vi "Wrap iPerf Test.vi"(7 "DUT Settings Ref":refnum<vi>, 8 "error in":errorcluster, 10 "iPerf Test Parameters":T2={"CLIENT iPERF PORT"=61000, "Protocol"=enum."TCP", "Force traffic (UDP only)"=enum."1M", "DURATION iPERF TEST (s)"=10, "Stack mode"=enum."IP stack"}, 11 "Client_adapter_IP_remote":string) -> (0 "error out":errorcluster, 2 "Server results":T1, 3 "Client results":T1)   [LabVIEW 2026]
uses:
  emea-tra-iPerf_bus_load_test/support/iperf3.Results.ctl
  emea-tra-iPerf_bus_load_test/support/iPerf_parameter.ctl
  emea-tra-iPerf_bus_load_test/support/iPerf_protocol.ctl
  emea-tra-iPerf_bus_load_test/support/bandwidth_selector.ctl
  emea-tra-iPerf_bus_load_test/support/Remote_test_info.ctl
  emea-tra-iPerf_bus_load_test/iPerfTest.lvlib
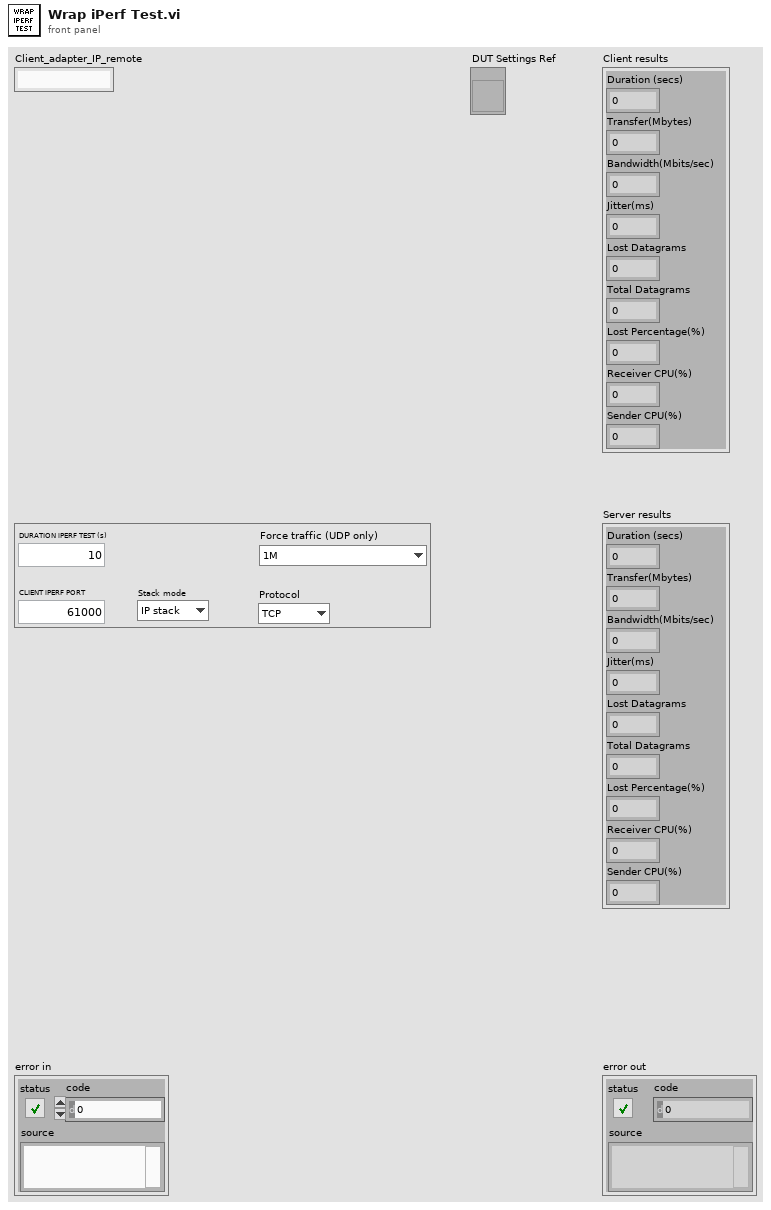
[diagram p1: front panel]
types:
  T1 = typedef "iPerfTest.lvlib/iperf3.Results.ctl" = cluster{"Duration (secs)":dbl, "Transfer(Mbytes)":dbl, "Bandwidth(Mbits/sec)":dbl, "Jitter(ms)":dbl, "Lost Datagrams":i32, "Total Datagrams":i32, "Lost Percentage(%)":dbl, "Receiver CPU(%)":dbl, "Sender CPU(%)":dbl}
  T2 = cluster{"CLIENT iPERF PORT":u16, "Protocol":enum16{"UDP", "TCP"}, "Force traffic (UDP only)":enum16{"1M", "10M", "20M", "30M", "40M", "50M", "100M", "500M", "1000M"}, "DURATION iPERF TEST (s)":u16, "Stack mode":enum16{"OS stack", "IP stack"}}
  T3 = typedef "iPerfTest.lvlib/Remote_test_info.ctl" = cluster{"PuTTY root folder ":path, "Remote Account Username":string, "Remote Account Password":string, "Server_adapter_IP_remote":string, "Client_adapter_IP_remote":string, "iPerf_path_remote_server":path, "iPerf_path_remote_client":path}
  T4 = typedef "iPerf_parameter.ctl" = cluster{"iPerf sending duration":i32, "Protocol":T5, "Force traffic (UDP only)":T6, "Port server":i32, "Port client":i32, "Stack mode":enum16{"OS stack", "IP stack"}}
  T5 = typedef "iPerf_protocol.ctl" = enum16{"UDP", "TCP"}
  T6 = typedef "bandwidth_selector.ctl" = enum16{"1M", "10M", "20M", "30M", "40M", "50M", "100M", "500M", "1000M"}
  T7 = enum16{"1M", "10M", "20M", "30M", "40M", "50M", "100M", "500M", "1000M"}
  T8 = typedef "DUT Info.ctl" = cluster{"DUT IP":string, "DUT Username":string, "DUT Password":string, "DUT SSH PORT":u16, "DUT FWD TEST PORT":u16, "DUT MAC ADDRESS":string}
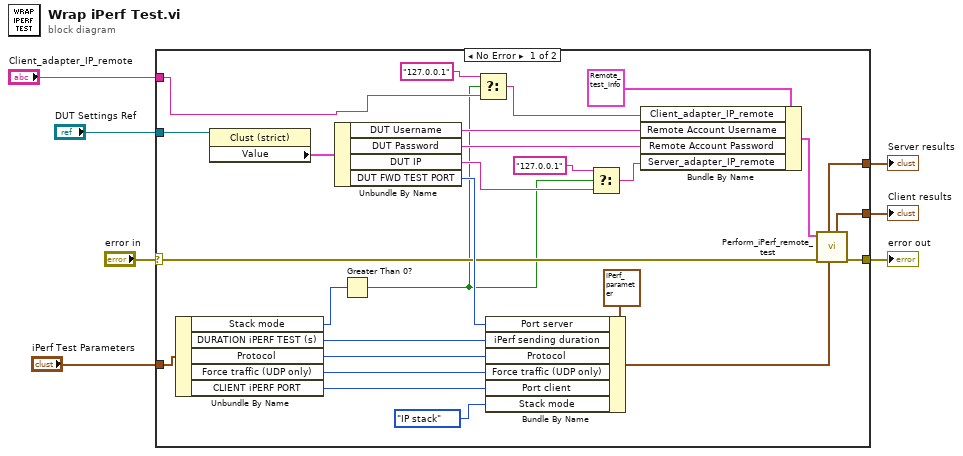
[diagram p0: block diagram]
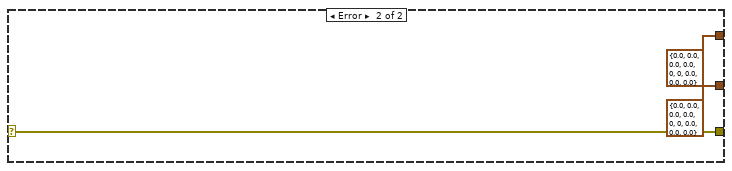
[diagram p2: hidden frame]
diagram:
  n1 = case shown="No Error" "error in" {
    selector: "error in" -> [w16 w35]
    tunnel: [w32 w35] -> w7
    tunnel: "DUT Settings Ref" -> [w30 _]
    tunnel: "iPerf Test Parameters" -> [w26 _]
    tunnel: [w18 T1 {"Duration (secs)"=0.0, "Transfer(Mbytes)"=0.0, "Bandwidth(Mbits/sec)"=0.0, "Jitter(ms)"=0.0, "Lost Datagrams"=0, "Total Datagrams"=0, "Lost Percentage(%)"=0.0, "Receiver CPU(%)"=0.0, "Sender CPU(%)"=0.0} ("Client results")] -> w4
    tunnel: [w17 T1 {"Duration (secs)"=0.0, "Transfer(Mbytes)"=0.0, "Bandwidth(Mbits/sec)"=0.0, "Jitter(ms)"=0.0, "Lost Datagrams"=0, "Total Datagrams"=0, "Lost Percentage(%)"=0.0, "Receiver CPU(%)"=0.0, "Sender CPU(%)"=0.0} ("Server results")] -> w3
    tunnel: "Client_adapter_IP_remote" -> [w10 _]
    frame No Error {
      n2 = Unbundle By Name(w26) -> ("Stack mode"=w12:enum16{"OS stack", "IP stack"}, "DURATION iPERF TEST (s)"=w25:u16, "Protocol"=w24:enum16{"UDP", "TCP"}, "Force traffic (UDP only)"=w23:T7, "CLIENT iPERF PORT"=w20:u16)
      n3 = property class="Clust (strict)"(reference=w30) -> ("Value"=w29:T8)  [unwired: 1 in, 2 out]
      n4 = Unbundle By Name(w29) -> ("DUT Username"=w28:string, "DUT Password"=w27:string, "DUT IP"=w13:string, "DUT FWD TEST PORT"=w22:u16)
      n5 = Greater Than 0?(x=w12) -> (x > 0?=w8:bool)
      n6 = Select(t="127.0.0.1" ("f"), s=w8, f=w10) -> (s? t:f=w9:string)
      n7 = Bundle By Name(cluster=T4 {"iPerf sending duration"=10, "Protocol"=enum."UDP", "Force traffic (UDP only)"=enum."1000M", "Port server"=0, "Port client"=0, "Stack mode"=enum."OS stack"} ("iPerf parameter"), "Port server"=w22, "iPerf sending duration"=w25, "Protocol"=w24, "Force traffic (UDP only)"=w23, "Port client"=w20, "Stack mode"=enum16{"OS stack", "IP stack"}."IP stack") -> (w19:T4)
      n8 = Select(t="127.0.0.1" ("f"), s=w8, f=w13) -> (s? t:f=w15:string)
      n9 = Bundle By Name(cluster=T3 {"PuTTY root folder "=path "C:/dev/emea-tra-iPerf_bus_load_test/utility/Putty_ssh_client", "Remote Account Username"="NI", "Remote Account Password"="123", "Server_adapter_IP_remote"="192.168.178.55", "Client_adapter_IP_remote"="192.168.178.51", "iPerf_path_remote_server"=path "C:/DEV/emea-tra-iPerf_bus_load_test/utility/iperf3.17.1_64", "iPerf_path_remote_client"=path "C:/DEV/emea-tra-iPerf_bus_load_test/utility/iperf3.17.1_64"} ("Remote test info"), "Client_adapter_IP_remote"=w9, "Remote Account Username"=w28, "Remote Account Password"=w27, "Server_adapter_IP_remote"=w15) -> (w34:T3)
      n10 = call "Perform_iPerf_remote_test.vi"("iPerf parameter"=w19, "error in (no error)"=w16, "Remote test info"=w34) -> ("error out"=w32:errorcluster, "Client results"=w18:T1, "Server results"=w17:T1)  [unwired: 4 in, 2 out]
    }
    frame Error {
    }
  }
  "error out" <- w7
  "Client results" <- w4
  "Server results" <- w3
